vi "ReadIni.vi"(1 "configuration file path":path=path "E:/LabVIEW/福尔达/AppData") -> ()   [LabVIEW 2018]
uses:
  <vilib>/Utility/config.llb/Read Key (Double).vi
  <vilib>/Utility/config.llb/Read Key (String).vi
  <vilib>/Utility/config.llb/Read Key (U32).vi
  <vilib>/Utility/config.llb/NI_LVConfig.lvlib
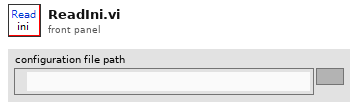
[diagram p1: front panel]
types:
  T1 = typedef "NI_LVConfig.lvlib/Config Data RefNum.ctl" = refnum<k1>
  T2 = cluster{"轮盘预压力":sgl, "泄漏量上限":sgl, "压力上限":sgl, "压力下限":sgl, "风门闭电压上限":sgl, "风门闭电压下限":sgl, "风门开电压上限":sgl, "风门开电压下限":sgl, "LED电流上限":sgl, "LED电流下限":sgl, "气压稳定时间":sgl, "伺服速度":sgl, "INV初始频率":sgl, "INV变化周期":sgl, "INV慢速变化量":sgl, "INV快速变化量":sgl}
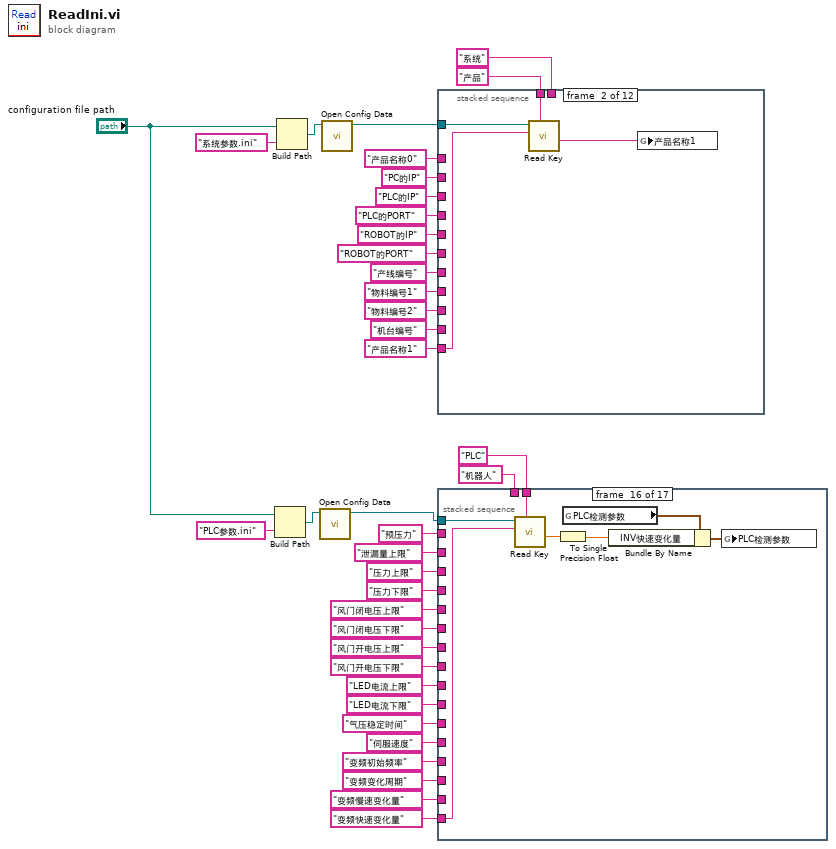
[diagram p0: block diagram]
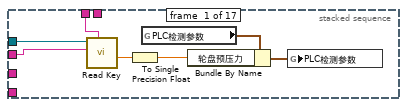
[diagram p2: hidden frame]
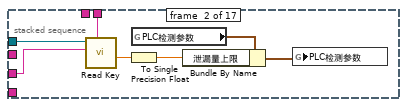
[diagram p3: hidden frame]
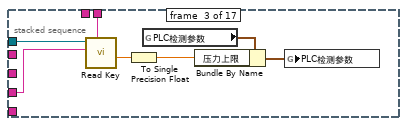
[diagram p4: hidden frame]
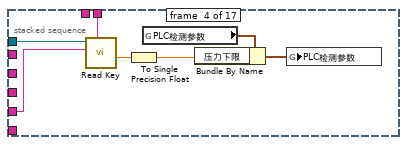
[diagram p5: hidden frame]
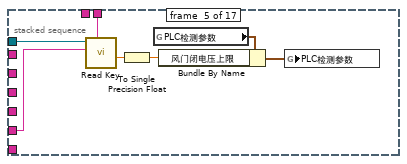
[diagram p6: hidden frame]
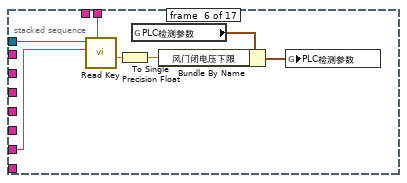
[diagram p7: hidden frame]
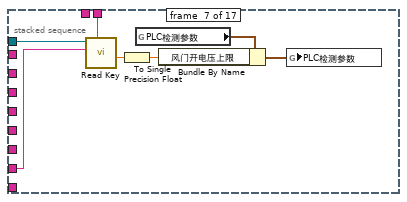
[diagram p8: hidden frame]
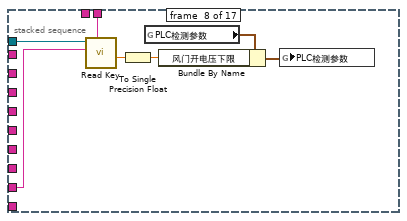
[diagram p9: hidden frame]
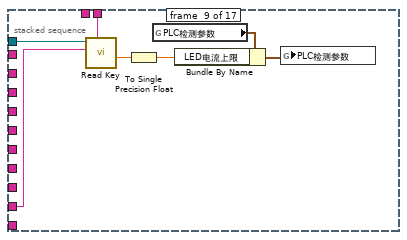
[diagram p10: hidden frame]
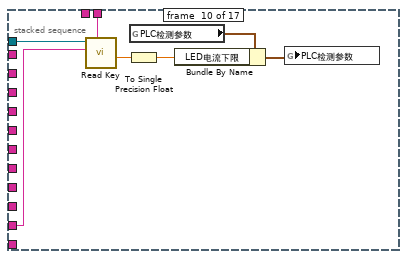
[diagram p11: hidden frame]
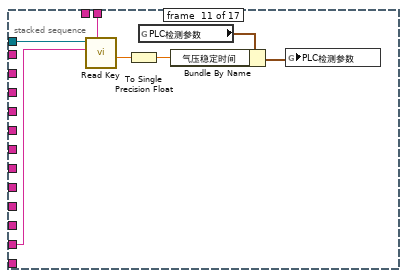
[diagram p12: hidden frame]
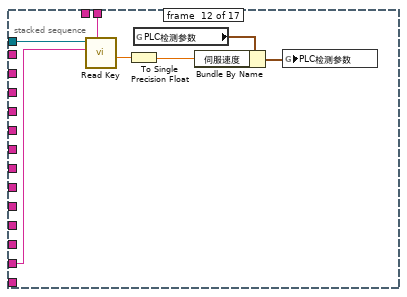
[diagram p13: hidden frame]
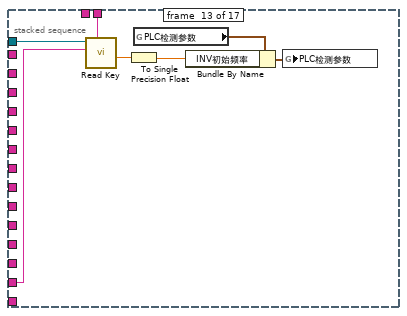
[diagram p14: hidden frame]
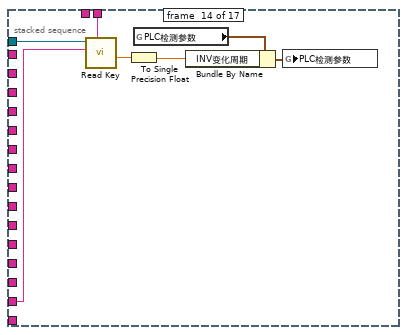
[diagram p15: hidden frame]
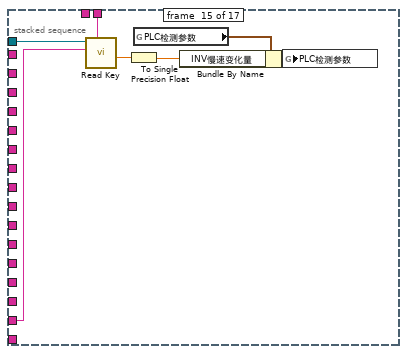
[diagram p16: hidden frame]
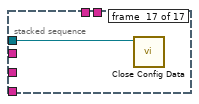
[diagram p17: hidden frame]
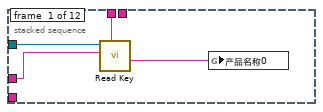
[diagram p18: hidden frame]
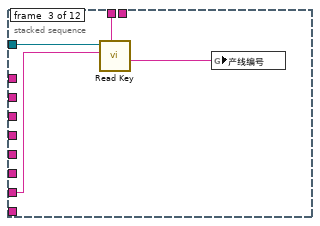
[diagram p19: hidden frame]
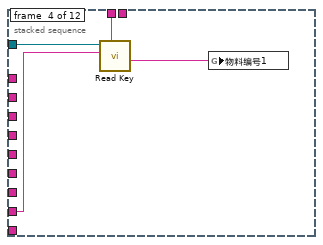
[diagram p20: hidden frame]
diagram:
  n1 = Build Path(base path="configuration file path", name or relative path="PLC参数.ini" ("名称或相对路径")) -> (appended path=w25:path)
  n2 = Build Path(base path="configuration file path", name or relative path="系统参数.ini" ("名称或相对路径")) -> (appended path=w38:path)
  n3 = call <vilib>:"Open Config Data.vi"("configuration file path"=w25) -> ("refnum"=w22:T1)  [unwired: 8 in, 2 out]
  n4 = call <vilib>:"Open Config Data.vi"("configuration file path"=w38) -> ("refnum"=w36:T1)  [unwired: 8 in, 2 out]
  n5 = stacked-sequence {
    tunnel: w36 -> [w41 w45 w49 w53 w57 w61 w65 w69 w73 w77 w81 w83]
    tunnel: "产品" -> [w40 w44 w48 w52 w56 w60 _ _ _ _ _ _]
    tunnel: "PC的IP" -> [_ _ _ _ _ _ w64 _ _ _ _ _]
    tunnel: "产品名称0" -> [w39 _ _ _ _ _ _ _ _ _ _ _]
    tunnel: "PLC的IP" -> [_ _ _ _ _ _ _ w68 _ _ _ _]
    tunnel: "PLC的PORT" -> [_ _ _ _ _ _ _ _ w72 _ _ _]
    tunnel: "ROBOT的IP" -> [_ _ _ _ _ _ _ _ _ w76 _ _]
    tunnel: "ROBOT的PORT" -> [_ _ _ _ _ _ _ _ _ _ w80 _]
    tunnel: "系统" -> [_ _ _ _ _ _ w63 w67 w71 w75 w79 _]
    tunnel: "产线编号" -> [_ _ w47 _ _ _ _ _ _ _ _ _]
    tunnel: "物料编号1" -> [_ _ _ w51 _ _ _ _ _ _ _ _]
    tunnel: "机台编号" -> [_ _ _ _ _ w59 _ _ _ _ _ _]
    tunnel: "物料编号2" -> [_ _ _ _ w55 _ _ _ _ _ _ _]
    tunnel: "产品名称1" -> [_ w43 _ _ _ _ _ _ _ _ _ _]
    frame #0 {
      n6 = call-poly <vilib>:"Read Key.vi"("section"=w40, "key"=w39, "refnum"=w41) -> ("value"=w42:string)  [unwired: 5 in, 3 out]
      n7 = global write "全局 1.vi" "产品名称0"(w42) -> ()
    }
    frame #1 {
      n8 = call-poly <vilib>:"Read Key.vi"("section"=w44, "key"=w43, "refnum"=w45) -> ("value"=w46:string)  [unwired: 5 in, 3 out]
      n9 = global write "全局 1.vi" "产品名称1"(w46) -> ()
    }
    frame #2 {
      n10 = call-poly <vilib>:"Read Key.vi"("section"=w48, "key"=w47, "refnum"=w49) -> ("value"=w50:string)  [unwired: 5 in, 3 out]
      n11 = global write "全局 1.vi" "产线编号"(w50) -> ()
    }
    frame #3 {
      n12 = call-poly <vilib>:"Read Key.vi"("section"=w52, "key"=w51, "refnum"=w53) -> ("value"=w54:string)  [unwired: 5 in, 3 out]
      n13 = global write "全局 1.vi" "物料编号1"(w54) -> ()
    }
    frame #4 {
      n14 = call-poly <vilib>:"Read Key.vi"("section"=w56, "key"=w55, "refnum"=w57) -> ("value"=w58:string)  [unwired: 5 in, 3 out]
      n15 = global write "全局 1.vi" "物料编号2"(w58) -> ()
    }
    frame #5 {
      n16 = call-poly <vilib>:"Read Key.vi"("section"=w60, "key"=w59, "refnum"=w61) -> ("value"=w62:string)  [unwired: 5 in, 3 out]
      n17 = global write "全局 1.vi" "机台编号"(w62) -> ()
    }
    frame #6 {
      n18 = call-poly <vilib>:"Read Key.vi"("section"=w63, "key"=w64, "refnum"=w65) -> ("value"=w66:string)  [unwired: 5 in, 3 out]
      n19 = global write "全局 1.vi" "CCIEFB Slave IP"(w66) -> ()
    }
    frame #7 {
      n20 = call-poly <vilib>:"Read Key.vi"("section"=w67, "key"=w68, "refnum"=w69) -> ("value"=w70:string)  [unwired: 5 in, 3 out]
      n21 = global write "全局 1.vi" "PLC IP"(w70) -> ()
    }
    frame #8 {
      n22 = call-poly <vilib>:"Read Key.vi"("section"=w71, "key"=w72, "refnum"=w73) -> ("value"=w74:u32)  [unwired: 5 in, 3 out]
      n23 = global write "全局 1.vi" "PLC PORT"(w74) -> ()
    }
    frame #9 {
      n24 = call-poly <vilib>:"Read Key.vi"("section"=w75, "key"=w76, "refnum"=w77) -> ("value"=w78:string)  [unwired: 5 in, 3 out]
      n25 = global write "全局 1.vi" "ROBOT IP"(w78) -> ()
    }
    frame #10 {
      n26 = call-poly <vilib>:"Read Key.vi"("section"=w79, "key"=w80, "refnum"=w81) -> ("value"=w82:u32)  [unwired: 5 in, 3 out]
      n27 = global write "全局 1.vi" "ROBOT PORT"(w82) -> ()
    }
    frame #11 {
      n28 = call <vilib>:"Close Config Data.vi"("refnum"=w83) -> ()  [unwired: 9 in, 2 out]
    }
  }
  n29 = stacked-sequence {
    tunnel: "机器人" -> [w86 _ _ _ _ _ _ _ _ _ _ _ _ _ _ _ _]
    tunnel: "PLC" -> [_ w93 w100 w107 w114 w121 w128 w135 w142 w149 w156 w163 w170 w177 w184 w191 _]
    tunnel: w22 -> [w85 w92 w99 w106 w113 w120 w127 w134 w141 w148 w155 w162 w169 w176 w183 w190 w196]
    tunnel: "预压力" -> [w84 _ _ _ _ _ _ _ _ _ _ _ _ _ _ _ _]
    tunnel: "泄漏量上限" -> [_ w91 _ _ _ _ _ _ _ _ _ _ _ _ _ _ _]
    tunnel: "压力上限" -> [_ _ w98 _ _ _ _ _ _ _ _ _ _ _ _ _ _]
    tunnel: "压力下限" -> [_ _ _ w105 _ _ _ _ _ _ _ _ _ _ _ _ _]
    tunnel: "风门闭电压上限" -> [_ _ _ _ w112 _ _ _ _ _ _ _ _ _ _ _ _]
    tunnel: "风门闭电压下限" -> [_ _ _ _ _ w119 _ _ _ _ _ _ _ _ _ _ _]
    tunnel: "风门开电压上限" -> [_ _ _ _ _ _ w126 _ _ _ _ _ _ _ _ _ _]
    tunnel: "风门开电压下限" -> [_ _ _ _ _ _ _ w133 _ _ _ _ _ _ _ _ _]
    tunnel: "LED电流上限" -> [_ _ _ _ _ _ _ _ w140 _ _ _ _ _ _ _ _]
    tunnel: "LED电流下限" -> [_ _ _ _ _ _ _ _ _ w147 _ _ _ _ _ _ _]
    tunnel: "气压稳定时间" -> [_ _ _ _ _ _ _ _ _ _ w154 _ _ _ _ _ _]
    tunnel: "伺服速度" -> [_ _ _ _ _ _ _ _ _ _ _ w161 _ _ _ _ _]
    tunnel: "变频初始频率" -> [_ _ _ _ _ _ _ _ _ _ _ _ w168 _ _ _ _]
    tunnel: "变频变化周期" -> [_ _ _ _ _ _ _ _ _ _ _ _ _ w175 _ _ _]
    tunnel: "变频慢速变化量" -> [_ _ _ _ _ _ _ _ _ _ _ _ _ _ w182 _ _]
    tunnel: "变频快速变化量" -> [_ _ _ _ _ _ _ _ _ _ _ _ _ _ _ w189 _]
    frame #0 {
      n30 = call-poly <vilib>:"Read Key.vi"("section"=w86, "key"=w84, "refnum"=w85) -> ("value"=w90:dbl)  [unwired: 5 in, 3 out]
      n31 = To Single Precision Float(number=w90) -> (single precision float=w89:sgl)
      n32 = global read "全局 1.vi" "PLC检测参数"() -> (w87:T2)
      n33 = Bundle By Name(cluster=w87, "轮盘预压力"=w89) -> (w88:T2)
      n34 = global write "全局 1.vi" "PLC检测参数"(w88) -> ()
    }
    frame #1 {
      n35 = call-poly <vilib>:"Read Key.vi"("section"=w93, "key"=w91, "refnum"=w92) -> ("value"=w97:dbl)  [unwired: 5 in, 3 out]
      n36 = To Single Precision Float(number=w97) -> (single precision float=w96:sgl)
      n37 = global read "全局 1.vi" "PLC检测参数"() -> (w94:T2)
      n38 = Bundle By Name(cluster=w94, "泄漏量上限"=w96) -> (w95:T2)
      n39 = global write "全局 1.vi" "PLC检测参数"(w95) -> ()
    }
    frame #2 {
      n40 = call-poly <vilib>:"Read Key.vi"("section"=w100, "key"=w98, "refnum"=w99) -> ("value"=w104:dbl)  [unwired: 5 in, 3 out]
      n41 = To Single Precision Float(number=w104) -> (single precision float=w103:sgl)
      n42 = global read "全局 1.vi" "PLC检测参数"() -> (w101:T2)
      n43 = Bundle By Name(cluster=w101, "压力上限"=w103) -> (w102:T2)
      n44 = global write "全局 1.vi" "PLC检测参数"(w102) -> ()
    }
    frame #3 {
      n45 = call-poly <vilib>:"Read Key.vi"("section"=w107, "key"=w105, "refnum"=w106) -> ("value"=w111:dbl)  [unwired: 5 in, 3 out]
      n46 = To Single Precision Float(number=w111) -> (single precision float=w110:sgl)
      n47 = global read "全局 1.vi" "PLC检测参数"() -> (w108:T2)
      n48 = Bundle By Name(cluster=w108, "压力下限"=w110) -> (w109:T2)
      n49 = global write "全局 1.vi" "PLC检测参数"(w109) -> ()
    }
    frame #4 {
      n50 = call-poly <vilib>:"Read Key.vi"("section"=w114, "key"=w112, "refnum"=w113) -> ("value"=w118:dbl)  [unwired: 5 in, 3 out]
      n51 = To Single Precision Float(number=w118) -> (single precision float=w117:sgl)
      n52 = global read "全局 1.vi" "PLC检测参数"() -> (w115:T2)
      n53 = Bundle By Name(cluster=w115, "风门闭电压上限"=w117) -> (w116:T2)
      n54 = global write "全局 1.vi" "PLC检测参数"(w116) -> ()
    }
    frame #5 {
      n55 = call-poly <vilib>:"Read Key.vi"("section"=w121, "key"=w119, "refnum"=w120) -> ("value"=w125:dbl)  [unwired: 5 in, 3 out]
      n56 = To Single Precision Float(number=w125) -> (single precision float=w124:sgl)
      n57 = global read "全局 1.vi" "PLC检测参数"() -> (w122:T2)
      n58 = Bundle By Name(cluster=w122, "风门闭电压下限"=w124) -> (w123:T2)
      n59 = global write "全局 1.vi" "PLC检测参数"(w123) -> ()
    }
    frame #6 {
      n60 = call-poly <vilib>:"Read Key.vi"("section"=w128, "key"=w126, "refnum"=w127) -> ("value"=w132:dbl)  [unwired: 5 in, 3 out]
      n61 = To Single Precision Float(number=w132) -> (single precision float=w131:sgl)
      n62 = global read "全局 1.vi" "PLC检测参数"() -> (w129:T2)
      n63 = Bundle By Name(cluster=w129, "风门开电压上限"=w131) -> (w130:T2)
      n64 = global write "全局 1.vi" "PLC检测参数"(w130) -> ()
    }
    frame #7 {
      n65 = call-poly <vilib>:"Read Key.vi"("section"=w135, "key"=w133, "refnum"=w134) -> ("value"=w139:dbl)  [unwired: 5 in, 3 out]
      n66 = To Single Precision Float(number=w139) -> (single precision float=w138:sgl)
      n67 = global read "全局 1.vi" "PLC检测参数"() -> (w136:T2)
      n68 = Bundle By Name(cluster=w136, "风门开电压下限"=w138) -> (w137:T2)
      n69 = global write "全局 1.vi" "PLC检测参数"(w137) -> ()
    }
    frame #8 {
      n70 = call-poly <vilib>:"Read Key.vi"("section"=w142, "key"=w140, "refnum"=w141) -> ("value"=w146:dbl)  [unwired: 5 in, 3 out]
      n71 = To Single Precision Float(number=w146) -> (single precision float=w145:sgl)
      n72 = global read "全局 1.vi" "PLC检测参数"() -> (w143:T2)
      n73 = Bundle By Name(cluster=w143, "LED电流上限"=w145) -> (w144:T2)
      n74 = global write "全局 1.vi" "PLC检测参数"(w144) -> ()
    }
    frame #9 {
      n75 = call-poly <vilib>:"Read Key.vi"("section"=w149, "key"=w147, "refnum"=w148) -> ("value"=w153:dbl)  [unwired: 5 in, 3 out]
      n76 = To Single Precision Float(number=w153) -> (single precision float=w152:sgl)
      n77 = global read "全局 1.vi" "PLC检测参数"() -> (w150:T2)
      n78 = Bundle By Name(cluster=w150, "LED电流下限"=w152) -> (w151:T2)
      n79 = global write "全局 1.vi" "PLC检测参数"(w151) -> ()
    }
    frame #10 {
      n80 = call-poly <vilib>:"Read Key.vi"("section"=w156, "key"=w154, "refnum"=w155) -> ("value"=w160:dbl)  [unwired: 5 in, 3 out]
      n81 = To Single Precision Float(number=w160) -> (single precision float=w159:sgl)
      n82 = global read "全局 1.vi" "PLC检测参数"() -> (w157:T2)
      n83 = Bundle By Name(cluster=w157, "气压稳定时间"=w159) -> (w158:T2)
      n84 = global write "全局 1.vi" "PLC检测参数"(w158) -> ()
    }
    frame #11 {
      n85 = call-poly <vilib>:"Read Key.vi"("section"=w163, "key"=w161, "refnum"=w162) -> ("value"=w167:dbl)  [unwired: 5 in, 3 out]
      n86 = To Single Precision Float(number=w167) -> (single precision float=w166:sgl)
      n87 = global read "全局 1.vi" "PLC检测参数"() -> (w164:T2)
      n88 = Bundle By Name(cluster=w164, "伺服速度"=w166) -> (w165:T2)
      n89 = global write "全局 1.vi" "PLC检测参数"(w165) -> ()
    }
    frame #12 {
      n90 = call-poly <vilib>:"Read Key.vi"("section"=w170, "key"=w168, "refnum"=w169) -> ("value"=w174:dbl)  [unwired: 5 in, 3 out]
      n91 = To Single Precision Float(number=w174) -> (single precision float=w173:sgl)
      n92 = global read "全局 1.vi" "PLC检测参数"() -> (w171:T2)
      n93 = Bundle By Name(cluster=w171, "INV初始频率"=w173) -> (w172:T2)
      n94 = global write "全局 1.vi" "PLC检测参数"(w172) -> ()
    }
    frame #13 {
      n95 = call-poly <vilib>:"Read Key.vi"("section"=w177, "key"=w175, "refnum"=w176) -> ("value"=w181:dbl)  [unwired: 5 in, 3 out]
      n96 = To Single Precision Float(number=w181) -> (single precision float=w180:sgl)
      n97 = global read "全局 1.vi" "PLC检测参数"() -> (w178:T2)
      n98 = Bundle By Name(cluster=w178, "INV变化周期"=w180) -> (w179:T2)
      n99 = global write "全局 1.vi" "PLC检测参数"(w179) -> ()
    }
    frame #14 {
      n100 = call-poly <vilib>:"Read Key.vi"("section"=w184, "key"=w182, "refnum"=w183) -> ("value"=w188:dbl)  [unwired: 5 in, 3 out]
      n101 = To Single Precision Float(number=w188) -> (single precision float=w187:sgl)
      n102 = global read "全局 1.vi" "PLC检测参数"() -> (w185:T2)
      n103 = Bundle By Name(cluster=w185, "INV慢速变化量"=w187) -> (w186:T2)
      n104 = global write "全局 1.vi" "PLC检测参数"(w186) -> ()
    }
    frame #15 {
      n105 = call-poly <vilib>:"Read Key.vi"("section"=w191, "key"=w189, "refnum"=w190) -> ("value"=w195:dbl)  [unwired: 5 in, 3 out]
      n106 = To Single Precision Float(number=w195) -> (single precision float=w194:sgl)
      n107 = global read "全局 1.vi" "PLC检测参数"() -> (w192:T2)
      n108 = Bundle By Name(cluster=w192, "INV快速变化量"=w194) -> (w193:T2)
      n109 = global write "全局 1.vi" "PLC检测参数"(w193) -> ()
    }
    frame #16 {
      n110 = call <vilib>:"Close Config Data.vi"("refnum"=w196) -> ()  [unwired: 9 in, 2 out]
    }
  }
